vi "LJU3_format_data.vi"(9 "value_array":dbl[](array[numeric]), 11 "time":timestamp) -> (0 "waveform_array_B":waveform(dbl)[](array[waveform])=[{"t0"=timestamp(0 s since 1904-01-01), "dt"=1.0, "Y"=[]}, {"t0"=timestamp(3732035173.078092 s since 1904-01-01), "dt"=1.0, "Y"=[302.8589782714844], "attributes"=variant("NI_ChannelName"=variant(string "T1"))}], 3 "waveform_array_A":waveform(dbl)[](array[waveform])=[{"t0"=timestamp(0 s since 1904-01-01), "dt"=1.0, "Y"=[]}, {"t0"=timestamp(3732035173.078092 s since 1904-01-01), "dt"=1.0, "Y"=[302.8589782714844], "attributes"=variant("NI_ChannelName"=variant(string "T1"))}])   [LabVIEW 2019]
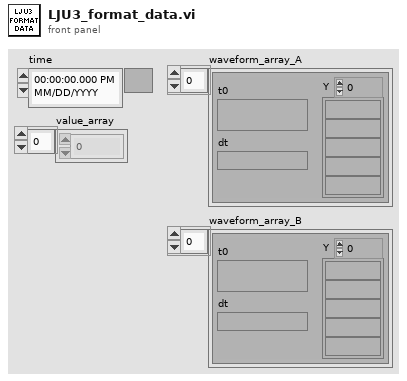
[diagram p1: front panel]
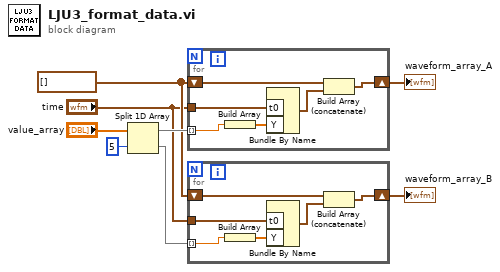
[diagram p0: block diagram]
diagram:
  w2 = waveform(dbl)[] []
  n1 = Split 1D Array(array="value_array", index=5) -> (first subarray=w5:dbl[], second subarray=w3:dbl[])
  n2 = for {
    tunnel: "time" -> [w12]
    tunnel: w5 -> [w10] mode=indexing
    shift-right: [w11] -> w8
    shift-left: w2 -> [w14]
    n3 = Build Array(w10) -> (w13:dbl[])
    n4 = Bundle By Name("t0"=w12, "Y"=w13) -> (w9:waveform(dbl))  [unwired: 1 in]
    n5 = Build Array (concatenate)(w14, w9) -> (w11:waveform(dbl)[])
  }
  "waveform_array_A" <- w8
  n6 = for {
    tunnel: "time" -> [w18]
    tunnel: w3 -> [w16] mode=indexing
    shift-right: [w17] -> w4
    shift-left: w2 -> [w20]
    n7 = Build Array(w16) -> (w19:dbl[])
    n8 = Bundle By Name("t0"=w18, "Y"=w19) -> (w15:waveform(dbl))  [unwired: 1 in]
    n9 = Build Array (concatenate)(w20, w15) -> (w17:waveform(dbl)[])
  }
  "waveform_array_B" <- w4
